vi "Write Fast FPGA Telem to FIFO.vi"   [LabVIEW 2014]
uses:
  FPGA Telem for Fast Logging.ctl
  <vilib>/FPGAPlugInAG/Dynamic/niLvFpga_Close_Dynamic.vi
  <vilib>/rvi/errors/niLvFpgaAdjustHostInterfaceError.vi
  <vilib>/Utility/error.llb/Error Cluster From Error Code.vi
  Global Data.vi
  <vilib>/rvi/interface/common/dynamic/niFpgaDynamicAddResources.vi
  <vilib>/FPGAPlugInAG/sbRIO-9626/niLvFpga_Open_sbRIO-9626.vi
  <vilib>/rvi/interface/nirviCloseFPGA/nirviCloseFPGA.xnode
  <vilib>/rvi/interface/nirviReadWriteControl/nirviReadWriteControl.xnode
  <vilib>/rvi/interface/nirviOpenFPGA/nirviOpenFPGA.xnode
  FPGA Bitfiles/FormulaElectric2_FPGATarget_FPGA_8a5J0mMac2U.lvbitx
  FPGA/Sensor Library/FPGA.vi
  NiFpgaLv.dll
  <vilib>/rvi/interface/Simulation/niFpgaSimulationCallBeginRW.vi
types:
  T1 = typedef "FPGA Telem for Fast Logging.ctl" = cluster{"Throttle 1 (V)":fxp<+/-,24,5>, "Throttle 2 (V)":fxp<+/-,24,5>, "Throttle 1 (%)":fxp<+/-,27,18>, "Throttle 2 (%)":fxp<+/-,27,18>, "Front BP (psi)":fxp<+/-,27,16>, "Rear BP (psi)":fxp<+/-,27,16>, "Front BP (V)":fxp<+/-,24,5>, "Rear BP (V)":fxp<+/-,24,5>, "Time Stamp":timestamp, "Accel X":dbl, "Accel Y":dbl, "Accel Z":dbl, "Gyro X":dbl, "Gyro Y":dbl, "Gyro Z":dbl}
  T2 = cluster{"read mode":enum16{"polling", "blocking"}, "write mode":enum16{"polling", "blocking"}}
  T3 = cluster{"Accel X":dbl, "Accel Y":dbl, "Accel Z":dbl, "Gyro X":dbl, "Gyro Y":dbl, "Gyro Z":dbl}
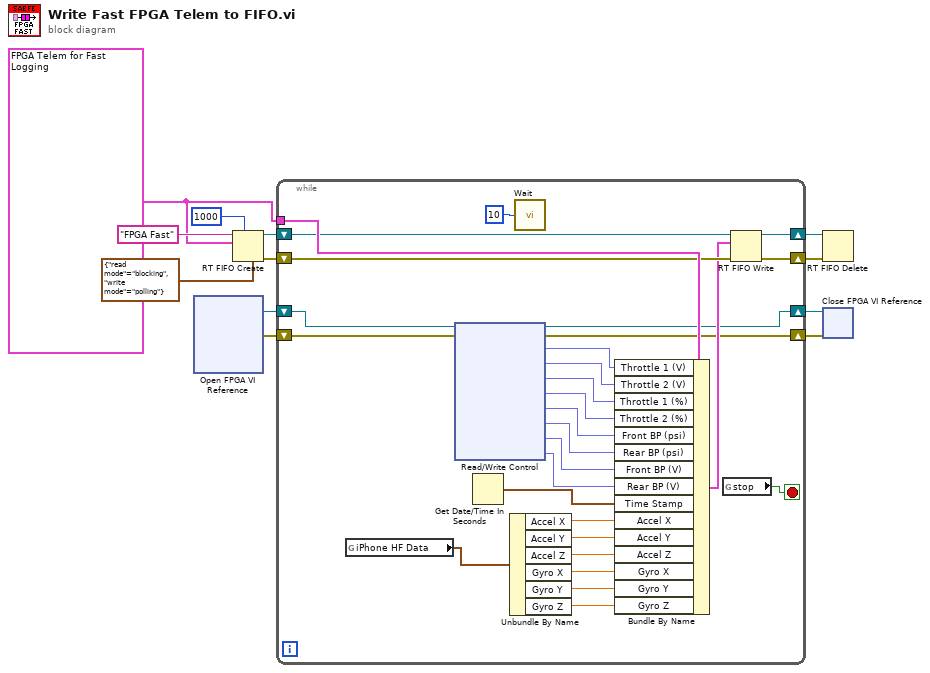
[diagram p0: block diagram]
diagram:
  w1 = T1 {"Throttle 1 (V)"=0.4218330383300781, "Throttle 2 (V)"=0.6996517181396484, "Throttle 1 (%)"=0.0, "Throttle 2 (%)"=0.0078125, "Front BP (psi)"=186.34033203125, "Rear BP (psi)"=185.44775390625, "Front BP (V)"=0.4808177947998047, "Rear BP (V)"=0.4820976257324219, "Time Stamp"=timestamp(0 s since 1904-01-01), "Accel X"=0.0, "Accel Y"=0.0, "Accel Z"=0.0, "Gyro X"=0.0, "Gyro Y"=0.0, "Gyro Z"=0.0} ("FPGA Fast Telem")
  n1 = xnode "Open FPGA VI Reference"() -> ("FPGA VI Reference Out"=w12:refnum<k20>, "error out"=w11:errorcluster)  [unwired: 2 in]
  n2 = RT FIFO Create(0:"FPGA Fast" ("name (unnamed)"), 1:w1, 4:u32 1000 ("size (10)"), 7:T2 {"read mode"=enum."blocking", "write mode"=enum."polling"} ("r/w modes (polling,polling)")) -> (8:w7:refnum<k33>, 11:w6:errorcluster)  [unwired: 4 in, 1 out]
  n3 = while {
    tunnel: w1 -> [w40]
    shift-right: [w33] -> w4
    shift-left: w7 -> [w36]
    shift-right: [w32] -> w5
    shift-left: w6 -> [w35]
    shift-right: [w30] -> w3
    shift-left: w12 -> [w38]
    shift-right: [w29] -> w2
    shift-left: w11 -> [w37]
    stop <- w39 stop-if-true
    n4 = global read "Global Data.vi" "iPhone HF Data"() -> (w19:T3)
    n5 = xnode "Read/Write Control"("FPGA VI Reference In"=w38, "error in"=w37) -> ("FPGA VI Reference Out"=w30:refnum<k20>, "error out"=w29:errorcluster, "Throttle 1 (V)"=w28:fxp<+/-,24,5>, "Throttle 2 (V)"=w27:fxp<+/-,24,5>, "Throttle 1 (%)"=w26:fxp<+/-,27,18>, "Throttle 2 (%)"=w25:fxp<+/-,27,18>, "Front BP (psi)"=w24:fxp<+,26,13>, "Rear BP (psi)"=w23:fxp<+,26,13>, "Front BP (V)"=w22:fxp<+/-,24,5>, "Rear BP (V)"=w21:fxp<+/-,24,5>)
    n6 = Get Date/Time In Seconds() -> (seconds since 1Jan1904=w20:timestamp)
    n7 = Unbundle By Name(w19) -> ("Accel X"=w18:dbl, "Accel Y"=w17:dbl, "Accel Z"=w16:dbl, "Gyro X"=w15:dbl, "Gyro Y"=w14:dbl, "Gyro Z"=w13:dbl)
    n8 = call "Wait"("Count(mSec)"=u32 10) -> ()  [unwired: 1 out]
    n9 = Bundle By Name(cluster=w40, "Throttle 1 (V)"=w28, "Throttle 2 (V)"=w27, "Throttle 1 (%)"=w26, "Throttle 2 (%)"=w25, "Front BP (psi)"=w24, "Rear BP (psi)"=w23, "Front BP (V)"=w22, "Rear BP (V)"=w21, "Time Stamp"=w20, "Accel X"=w18, "Accel Y"=w17, "Accel Z"=w16, "Gyro X"=w15, "Gyro Y"=w14, "Gyro Z"=w13) -> (w34:T1)
    n10 = global read "Global Data.vi" "stop"() -> (w39:bool)
    n11 = RT FIFO Write(0:w36, 1:w34, 3:w35) -> (8:w33:refnum<k33>, 11:w32:errorcluster)  [unwired: 2 in, 2 out]
  }
  n12 = RT FIFO Delete(0:w4, 3:w5) -> ()  [unwired: 1 in, 1 out]
  n13 = xnode "Close FPGA VI Reference"("FPGA VI Reference In"=w3, "error in"=w2) -> ()  [unwired: 1 out]
